vi "Read Earthed.vi"(4 "error in":errorcluster) -> (0 "error out":errorcluster, 2 "Dump Switch mimic":bool)   [LabVIEW 2015]
uses:
  <vilib>/DAQmx/read.llb/DAQmx Read (Digital Bool 1Line 1Point).vi
  <vilib>/DAQmx/write.llb/DAQmx Write (Digital Bool 1Line 1Point).vi
  <vilib>/DAQmx/miscellaneous.llb/DAQmx Fill In Error Info.vi
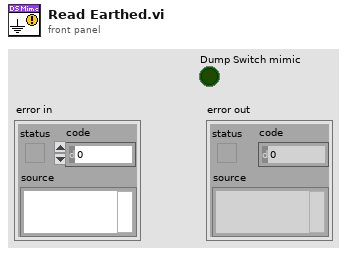
[diagram p1: front panel]
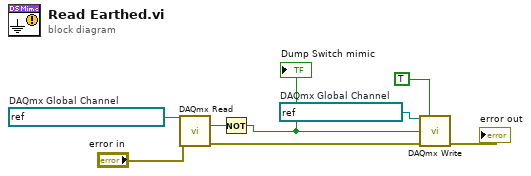
[diagram p0: block diagram]
diagram:
  w4 = refnum<k21> "DO11 Earthed LED"  # DAQmx Global Channel
  w5 = refnum<k21> "DI5 Dump Switch mimic"  # DAQmx Global Channel
  n1 = call-poly <vilib>:"DAQmx Read.vi"("task/channels in"=w5, "error in"="error in") -> ("data"=w7:bool, "error out"=w8:errorcluster)  [unwired: 11 in, 1 out]
  n2 = Not(x=w7) -> (.not. x?=w6:bool)
  "Dump Switch mimic" <- w6
  n3 = call-poly <vilib>:"DAQmx Write.vi"("task/channels in"=w4, "auto start"=TRUE, "data"=w6, "error in"=w8) -> ("error out"=→"error out":errorcluster)  [unwired: 9 in, 2 out]
